vi "Default Channel Configuration.vi"() -> (2 "Conversion Time":u32(ring) items=["200 ms", "2.5 ms"], 3 "Degree Range":u32(ring)=2 items=["Raw Ohms", "Degrees Kelvin", "Degrees Celsius", "Degrees Fahrenheit", "Degrees Rankine"], 4 "RTD type":T1=2 items=["User Defined"=0, "TCR3750"=2, "TCR3851"=7], 6 "RTD_A":dbl=0.0039083, 8 "RTD_B":dbl=-5.775e-07, 10 "RTD_C":dbl=-4.183e-12, 15 "RTD_Ro":dbl=100.0)   [LabVIEW 2017, in "Modules.lvlib" / "9226.lvclass"]
uses:
  9226.lvclass
  Supported RTD Types.ctl
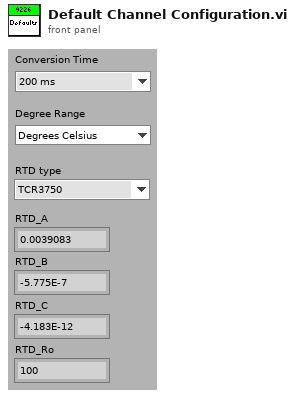
[diagram p1: front panel]
types:
  T1 = typedef "Modules.lvlib/9226.lvclass/Supported RTD Types.ctl" = u32
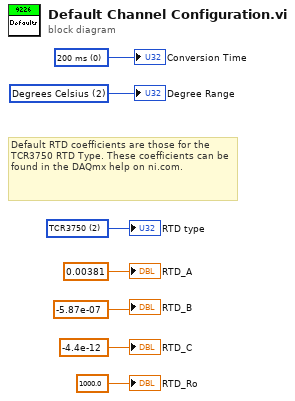
[diagram p0: block diagram]
diagram:
  w1 = T1 2 items=["User Defined"=0, "TCR3750"=2, "TCR3851"=7] ("RTD type")
  w2 = u32 2 items=["Raw Ohms", "Degrees Kelvin", "Degrees Celsius", "Degrees Fahrenheit", "Degrees Rankine"] ("Temperature Units")
  w3 = u32 0 items=["200 ms", "2.5 ms"] ("Conversion Time")
  # "Default RTD coefficients are those for the TCR3750 RTD Type. These coefficients can be found in the DAQmx help on ni.com."
  "RTD_A" <- 0.00381 ("Numeric")
  "RTD_B" <- -5.87e-07 ("Numeric")
  "RTD_C" <- -4.4e-12 ("Numeric")
  "RTD_Ro" <- 1000.0 ("Numeric")
  "Conversion Time" <- w3
  "Degree Range" <- w2
  "RTD type" <- w1
